vi "Init b.vi"(0 "connection ID in":refnum<k31>, 2 "Board Type (Uno)":T1, 3 "Bytes Per Packet (15)":u32=15, 4 "Connection Type (USB/Serial)":T2, 5 "error in":errorcluster) -> (14 "Arduino Resource out":T3, 19 "error out":errorcluster)   [LabVIEW 2015]
doc: "Initializes a connection to an Arduino running the LabVIEW Interface for Arduino sketch.\n\nNote: The baud rate specified must match the baud rate defined by DEFAULTBAUDRATE in the Arduino firmware.\n\nNote: The Bytes Per Packet input must match the COMMANDLENGTH specified in the Arduino firmware."
uses:
  <vilib>/LabVIEW Interface for Arduino/Type Defs/Board Type.ctl
  <vilib>/LabVIEW Interface for Arduino/Type Defs/Connection Type.ctl
  <vilib>/LabVIEW Interface for Arduino/LabVIEW Interface for Arduino.lvlib
panel:
  in  "MaxNumTimeouts (20)":u32=50
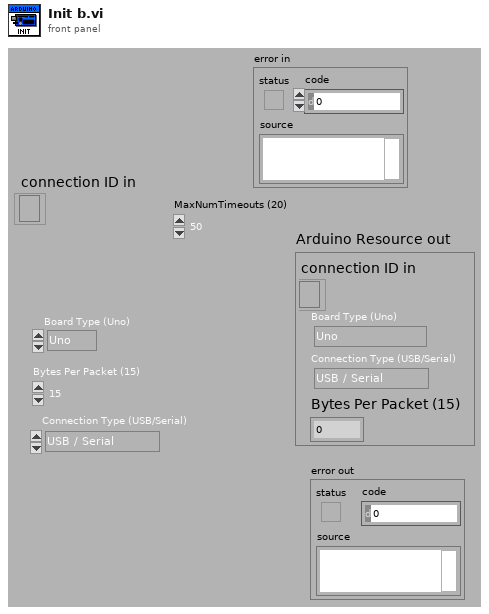
[diagram p1: front panel]
types:
  T1 = typedef "LabVIEW Interface for Arduino.lvlib/Board Type.ctl" = enum16{"Uno", "Dimuelanove w/Atmega 328", "Mega 2560"}
  T2 = typedef "LabVIEW Interface for Arduino.lvlib/Connection Type.ctl" = enum8{"USB / Serial", "XBEE", "BlueSmirf (Bluetooth)"}
  T3 = cluster{"connection ID in":refnum<k31>, "Board Type (Uno)":T1, "Connection Type (USB/Serial)":T2, "Bytes Per Packet (15)":u32}
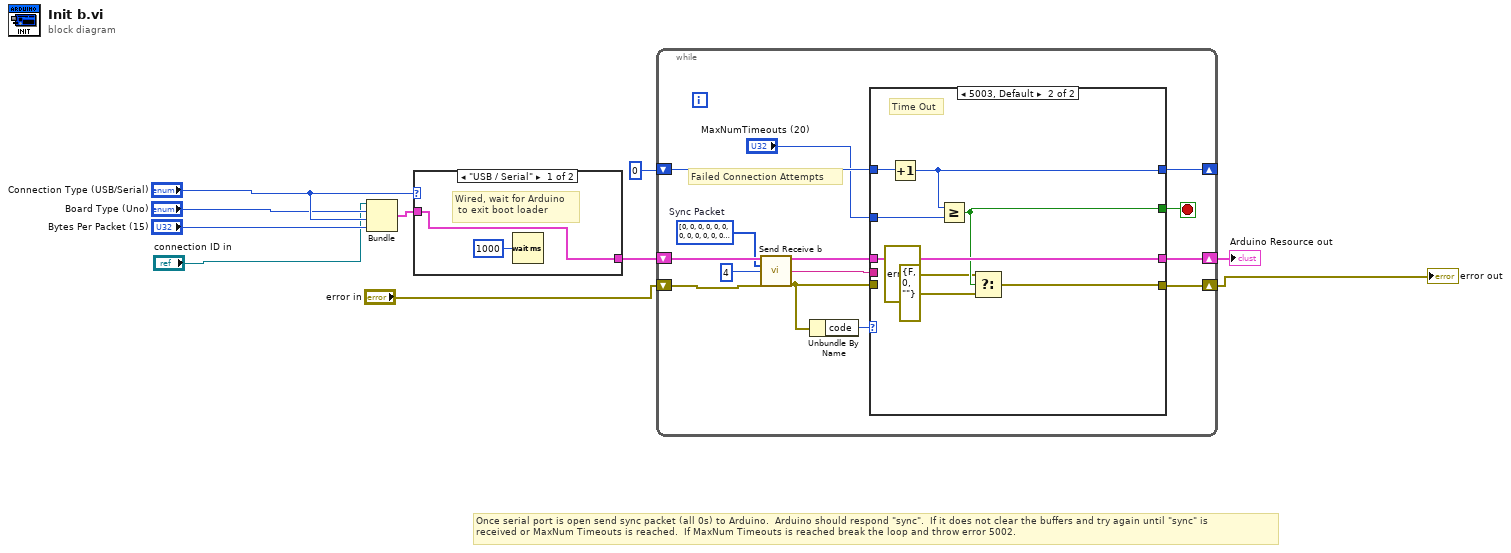
[diagram p0: block diagram]
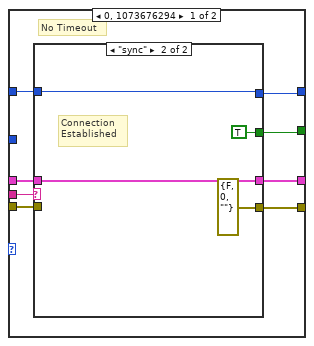
[diagram p3: hidden frame]
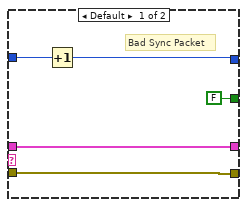
[diagram p4: hidden frame]
diagram:
  # "Once serial port is open send sync packet (all 0s) to Arduino.  Arduino should respond \"sync\".  If it does not clear the buffers and try again until \"sync\" is \nreceived or MaxNum Timeouts is reached.  If MaxNum Timeouts is reached break the loop and throw error 5002."
  n1 = Bundle("connection ID in"="connection ID in", "Board Type (Uno)"="Board Type (Uno)", "Connection Type (USB/Serial)"="Connection Type (USB/Serial)", "Bytes Per Packet (15)"="Bytes Per Packet (15)") -> (w4:T3)  [unwired: 1 in]
  n2 = case shown="\"USB / Serial\"" "Connection Type (USB/Serial)" {
    tunnel: w4 -> [w11 w13]
    tunnel: [w11 w13] -> w5
    frame "USB / Serial" {
      # "Wired, wait for Arduino\n to exit boot loader"
      n3 = Wait (ms)(milliseconds to wait=u32 1000) -> ()  [unwired: 1 out]
    }
    frame Default {
    }
  }
  n4 = while {
    shift-right: [w22] -> w2
    shift-left: w5 -> [w20]
    shift-right: [w23] -> w3
    shift-left: "error in" -> [w17]
    shift-right: [w26] -> _
    shift-left: 0 -> [w25]
    stop <- w24 stop-if-true
    w18 = u8[] [0, 0, 0, 0, 0, 0, 0, 0, 0, 0, 0, 0, 0]  # Sync Packet
    # "Failed Connection Attempts"
    n5 = call "Send Receive b.vi"("Arduino Resource"=w20, "Data"=w18, "Bytes To Read (0)"=u32 4, "error in"=w17) -> ("Arduino Resource out"=w16:T3, "Read Buffer"=w15:string, "error out"=w14:errorcluster)  [unwired: 9 in]
    n6 = Unbundle By Name(w14) -> ("code"=w27:i32)
    n7 = case shown="5003, Default" w27 {
      tunnel: [w31 w51] -> w26
      tunnel: w25 -> [w30 w52]
      tunnel: [w28 w49] -> w24
      tunnel: [w34 w45] -> w23
      tunnel: [w33 w50] -> w22
      tunnel: w16 -> [w32 w50]
      tunnel: w15 -> [w35 _]
      tunnel: w14 -> [w29 _]
      tunnel: "MaxNumTimeouts (20)" -> [_ w48]
      frame 0, 1073676294 {
        # "No Timeout"
        n8 = case shown="\"sync\"" w35 {
          tunnel: [w36 errorcluster {"status"=FALSE, "code"=0, "source"=""} ("error out")] -> w34
          tunnel: [w37 w43] -> w33
          tunnel: w32 -> [w37 w43]
          tunnel: [FALSE TRUE] -> w28
          tunnel: w30 -> [w39 w41]
          tunnel: [w38 w41] -> w31
          tunnel: w29 -> [w36 _]
          frame Default {
            # "Bad Sync Packet"
            n9 = Increment(x=w39) -> (x+1=w38:i32)
          }
          frame "sync" {
            # "Connection \nEstablished"
          }
        }
      }
      frame 5003, Default {
        # "Time Out"
        n10 = Increment(x=w52) -> (x+1=w51:i32)
        n11 = Greater Or Equal?(x=w51, y=w48) -> (x >= y?=w49:bool)
        n12 = Select(t=errorcluster {"status"=TRUE, "code"=5002, "source"="Init.vi.  Unable to establish connection with Arduino.  Please ensure that you have selected the correct COM port and that you have flashed the Arduino with the correct firmware."} ("error out"), s=w49, f=errorcluster {"status"=FALSE, "code"=0, "source"=""}) -> (s? t:f=w45:errorcluster)
      }
    }
  }
  "error out" <- w3
  "Arduino Resource out" <- w2
